vi "Initialize Master.vi"(8 "error in (no error)":errorcluster, 11 "network master in":refnum<class "Network Master.lvclass">) -> (0 "error out":errorcluster, 3 "network master out":refnum<class "Network Master.lvclass">)   [LabVIEW 2018, in "SubVIs.lvlib" / "Network Master.lvclass"]
doc: "This provides an interface for the master to open a connection to the slave."
uses:
  Network Master.lvclass
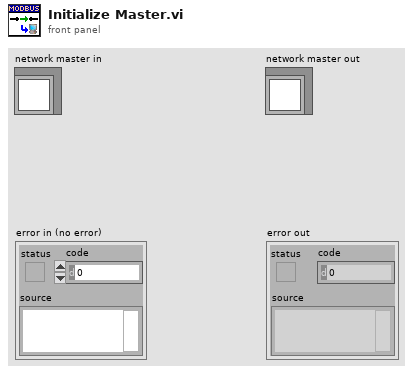
[diagram p1: front panel]
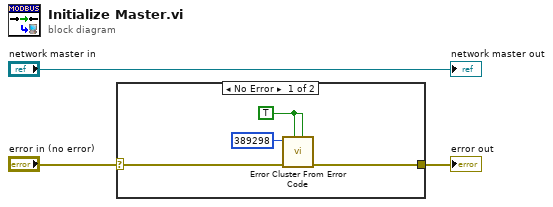
[diagram p0: block diagram]
diagram:
  n1 = case shown="No Error" "error in (no error)" {
    selector: "error in (no error)" -> [w6 w8]
    tunnel: [w7 w8] -> w1
    frame No Error {
      w4 = TRUE ("show call chain? (False)")
      n2 = call "Error Cluster From Error Code.vi"("is warning? (False)"=w4, "show call chain? (False)"=w4, "error in (no error)"=w6, "error code (0)"=389298) -> ("error out"=w7:errorcluster)  [unwired: 5 in]
    }
    frame Error {
    }
  }
  "error out" <- w1
  "network master out" <- "network master in"
